vi "Get settings chain.vi"(8 "error in (no error)":errorcluster, 11 "DAQMH121119OrcaFlashBase in":refnum<class "DAQOrcaFlash.lvclass">) -> (0 "error out":errorcluster, 1 "class name":string[](array[string]), 2 "settings":variant[](array[variant]), 3 "DAQMH121119OrcaFlashBase out":refnum<class "DAQOrcaFlash.lvclass">)   [LabVIEW 2012, in "DAQOrcaFlash.lvclass"]
doc: "Returns an array of variants containing the settings clusters of each class in the inheritance chain (lowest child class first), together with an array of all class names in the inheritance chain.\n\nFor classes without settings cluster, the settings chain contains empty variants."
uses:
  DAQOrcaFlash.lvclass
  <vilib>/Distrio/Murmex/Murmex/Murmex.lvclass
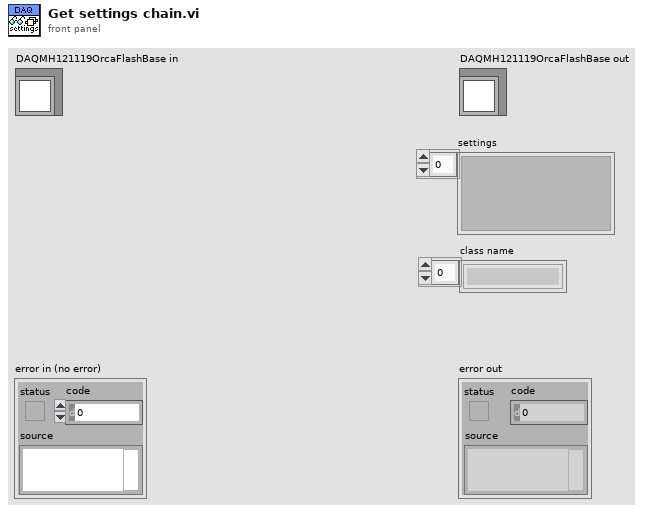
[diagram p1: front panel]
types:
  T1 = typedef "DAQOrcaFlash.lvclass/settings_cluster.ctl" = cluster{"no. of frames":i32, "imaging mode":T2, "exposure time":dbl[unit], "binning":T3, "x resolution":i32, "y resolution":i32, "x offset":i32, "y offset":i32, "Width of slit in image space ":dbl[unit], "number of pulses":i32, "Rolling shutter pace":sgl[unit], "Frames per second":dbl[unit], "Custom saving path":bool, "Subfolder levels":string[], "File name":string, "button:AO":bool, "Merit factor":dbl, "Merit factor type":T4, "Conversion policy":cluster{"Conversion Method":u32, "Minimum Value":i32, "Maximum Value":i32, "# Shifts":i32}, "wait b4 acquisition":dbl[unit]}
  T2 = typedef "DAQOrcaFlash.lvclass/imaging_mode.ctl" = enum16{"focus mode", "single sweep"}
  T3 = typedef "DAQOrcaFlash.lvclass/binning.ctl" = u16
  T4 = typedef "DAQOrcaFlash.lvclass/merit_factor_type.ctl" = enum16{"full frame intensity", "ROI beads", "Weber contrast", "Michelson contrast", "RMS contrast", "Line profile analysis", "ROI analysis", "FFT", "SNR", "5% brightest"}
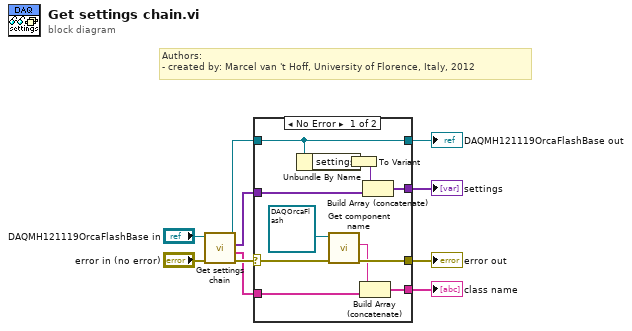
[diagram p0: block diagram]
diagram:
  # "Authors: \n- created by: Marcel van 't Hoff, University of Florence, Italy, 2012"
  n1 = call-parent "Get settings chain.vi"("error in (no error)"="error in (no error)", "MurmexBase in"="DAQMH121119OrcaFlashBase in") -> ("error out"=w8:errorcluster, "class name"=w5:string[], "settings"=w6:variant[], "MurmexBase out"=w7:refnum<class "DAQOrcaFlash.lvclass">)  [unwired: 6 in]
  n2 = case shown="No Error" w8 {
    selector: w8 -> [w21 w25]
    tunnel: [w20 w25] -> w1
    tunnel: [w11 w24] -> w3
    tunnel: w7 -> [w11 w24]
    tunnel: [w18 w23] -> w2
    tunnel: [w17 w22] -> w4
    tunnel: w6 -> [w13 w22]
    tunnel: w5 -> [w16 w23]
    frame No Error {
      n3 = Unbundle By Name(w11) -> ("settings"=w15:T1)
      n4 = call <vilib>:"Get component name.vi"("error in (no error)"=w21, "Murmex in"=refnum<class "DAQOrcaFlash.lvclass"> refnum ("DAQMH121119OrcaFlash.lvclass")) -> ("error out"=w20:errorcluster, "component name"=w19:string)  [unwired: 7 in, 1 out]
      n5 = To Variant(anything=w15) -> (Variant=w14:variant)
      n6 = Build Array (concatenate)(w19, w16) -> (w18:string[])
      n7 = Build Array (concatenate)(w14, w13) -> (w17:variant[])
    }
    frame Error {
    }
  }
  "error out" <- w1
  "DAQMH121119OrcaFlashBase out" <- w3
  "settings" <- w4
  "class name" <- w2
